vi "连接数据库.vi"(8 "error in (no error)":errorcluster) -> (0 "error out":errorcluster, 3 "ADODB._Connection Out":refnum<k7>)   [LabVIEW 2013]
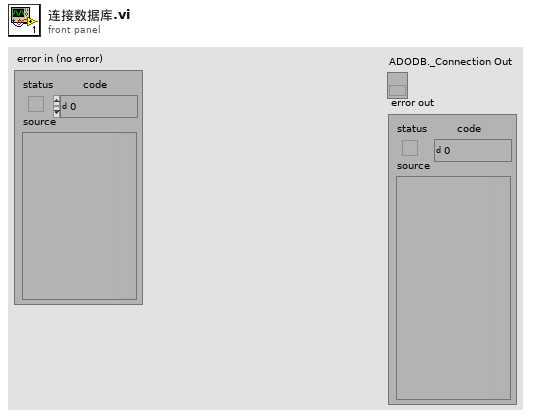
[diagram p1: front panel]
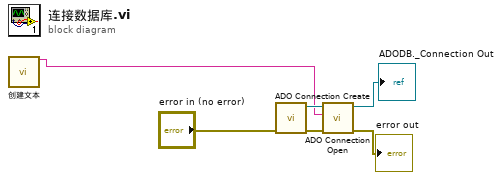
[diagram p0: block diagram]
diagram:
  n1 = call "创建文本"() -> ("Result"=w1:string)  [unwired: 14 in, 1 out]
  n2 = call "ADO Connection Create.vi"("error in (no error)"="error in (no error)") -> ("error out"=w5:errorcluster, "ADODB._Connection Out"=w6:refnum<k7>)  [unwired: 9 out]
  n3 = call "ADO Connection Open.vi"("error in (no error)"=w5, "ConnectionString"=w1, "ADODB._Connection In"=w6) -> ("error out"=→"error out":errorcluster, "ADODB._Connection Out"=→"ADODB._Connection Out":refnum<k7>)  [unwired: 7 out]
